vi "Data available.vi"(8 "error in":errorcluster, 10 "Data":string, 11 "Module ID":i32=-1) -> (0 "error out":errorcluster)   [LabVIEW 2020, in "Arduino stepper.lvlib"]
doc: "Broadcast a message whenever data is present at the input port.\n_____\nCreated using DQMH Event Scripter 6.1.0.128."
uses:
  Arduino stepper.lvlib
  Data available Argument--cluster.ctl
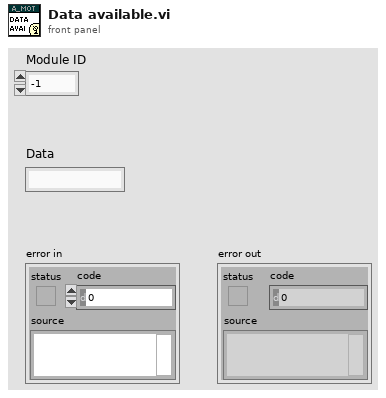
[diagram p1: front panel]
types:
  T1 = typedef "Arduino stepper.lvlib/Data available Argument--cluster.ctl" = cluster{"Module ID":i32, "Data":string}
  T2 = typedef "Arduino stepper.lvlib/Broadcast Events--cluster.ctl" = cluster{"Module Did Init":refnum<user-event>, "Status Updated":refnum<user-event>, "Error Reported":refnum<user-event>, "Module Did Stop":refnum<user-event>, "Update Module Execution Status":refnum<user-event>, "Device connected":refnum<user-event>, "Data available":refnum<user-event>}
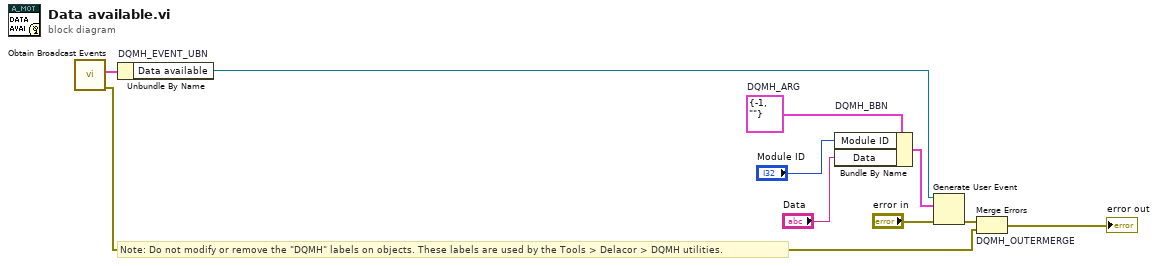
[diagram p0: block diagram]
diagram:
  w5 = T1 {"Module ID"=-1, "Data"=""}  # DQMH_ARG
  # "Note: Do not modify or remove the \"DQMH\" labels on objects. These labels are used by the Tools > Delacor > DQMH utilities."
  n1 = call "Obtain Broadcast Events.vi"() -> ("error out"=w2:errorcluster, "Arduino stepper Broadcast Events"=w1:T2)  [unwired: 10 in]
  n2 = Unbundle By Name "DQMH_EVENT_UBN"(w1) -> ("Data available"=w7:refnum<user-event>)
  n3 = Bundle By Name "DQMH_BBN"(cluster=w5, "Module ID"="Module ID", "Data"="Data") -> (w8:T1)
  n4 = Generate User Event(user event=w7, event data cluster=w8, error in="error in") -> (error out=w6:errorcluster)  [unwired: 1 in, 1 out]
  n5 = Merge Errors "DQMH_OUTERMERGE"(w6, w2) -> (→"error out":errorcluster)
